vi "Get ESP System Configuration.vi"(4 "error in (no error)":errorcluster, 7 "VISA resource name":refnum<visa-resource-name>) -> (0 "error out":errorcluster, 2 "ESP system Configuration":T1, 3 "VISA resource name out":refnum<visa-resource-name>)   [LabVIEW 2014, in "Newport ESP301.lvlib"]
doc: "This command is used to get the present ESP system stage/driver configuration. After each system reset or initialization the ESP motion controller detects the presence of Universal drivers and ESP-compatible stages connected."
uses:
  Newport ESP301.lvlib
panel:
  # "Axis 2 ESP compatible motorized positionner detected"
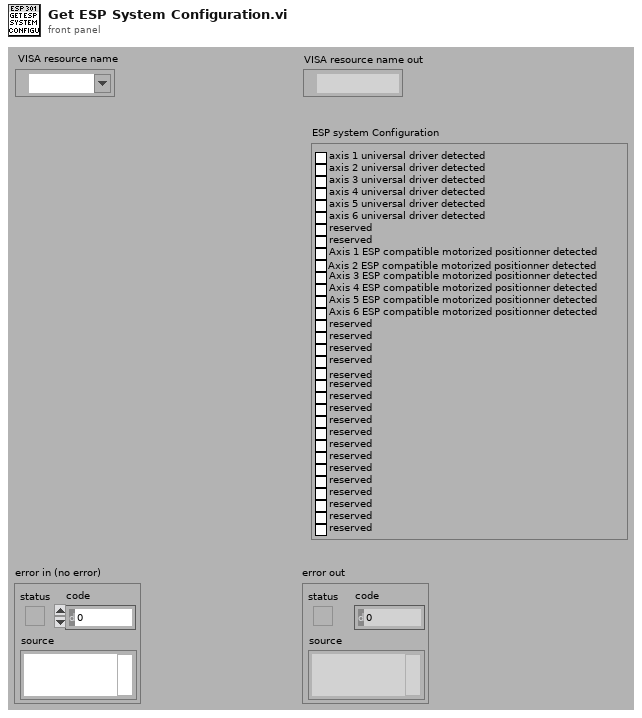
[diagram p1: front panel]
types:
  T1 = cluster{"axis 1 universal driver detected":bool, "axis 2 universal driver detected":bool, "axis 3 universal driver detected":bool, "axis 4 universal driver detected":bool, "axis 5 universal driver detected":bool, "axis 6 universal driver detected  ":bool, "reserved":bool, "reserved":bool, "Axis 1 ESP compatible motorized positionner detected  ":bool, bool, "Axis 3 ESP compatible motorized positionner detected  ":bool, "Axis 4 ESP compatible motorized positionner detected  ":bool, "Axis 5 ESP compatible motorized positionner detected   ":bool, "Axis 6 ESP compatible motorized positionner detected   ":bool, "reserved":bool, "reserved ":bool, "reserved":bool, "reserved ":bool, "reserved ":bool, "reserved ":bool, "reserved ":bool, "reserved ":bool, "reserved ":bool, "reserved ":bool, "reserved ":bool, "reserved ":bool, "reserved ":bool, "reserved ":bool, "reserved ":bool, "reserved ":bool, "reserved ":bool, "reserved":bool}
  T2 = cluster{"Boolean array[0]":bool, "Boolean array[1]":bool, "Boolean array[2]":bool, "Boolean array[3]":bool, "Boolean array[4]":bool, "Boolean array[5]":bool, "Boolean array[6]":bool, "Boolean array[7]":bool, "Boolean array[8]":bool, "Boolean array[9]":bool, "Boolean array[10]":bool, "Boolean array[11]":bool, "Boolean array[12]":bool, "Boolean array[13]":bool, "Boolean array[14]":bool, "Boolean array[15]":bool, "Boolean array[16]":bool, "Boolean array[17]":bool, "Boolean array[18]":bool, "Boolean array[19]":bool, "Boolean array[20]":bool, "Boolean array[21]":bool, "Boolean array[22]":bool, "Boolean array[23]":bool, "Boolean array[24]":bool, "Boolean array[25]":bool, "Boolean array[26]":bool, "Boolean array[27]":bool, "Boolean array[28]":bool, "Boolean array[29]":bool, "Boolean array[30]":bool, "Boolean array[31]":bool}
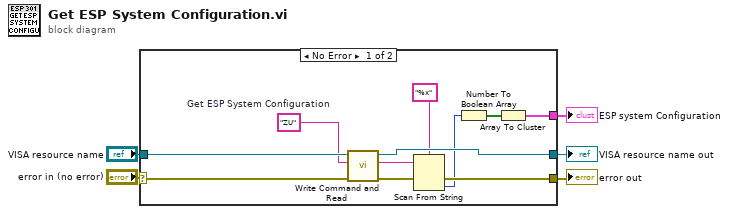
[diagram p0: block diagram]
diagram:
  n1 = case shown="No Error" "error in (no error)" {
    selector: "error in (no error)" -> [w14 w18]
    tunnel: [w9 w18] -> w5
    tunnel: "VISA resource name" -> [w16 w17]
    tunnel: [w15 w17] -> w4
    tunnel: [w8 _] -> w1
    frame No Error {
      w13 = "ZU"  # Get ESP System Configuration
      n2 = call "Write Command and Read.vi"("error in (no error)"=w14, "Command"=w13, "VISA resource name"=w16) -> ("error out"=w10:errorcluster, "Returned string"=w6:string, "VISA resource name out"=w15:refnum<visa-resource-name>)  [unwired: 2 in, 2 out]
      n3 = Scan From String(format string="%x" ("chaîne de format"), input string=w6, error in=w10) -> (error out=w9:errorcluster, output 1=w7:u32)  [unwired: 2 in, 2 out]
      n4 = Number To Boolean Array(number=w7) -> (Boolean array=w12:bool[])
      n5 = Array To Cluster(array=w12) -> (cluster=w8:T2)
    }
    frame Error {
    }
  }
  "error out" <- w5
  "VISA resource name out" <- w4
  "ESP system Configuration" <- w1
